vi "S2DS_Edit Channel Info.vi"(4 "error in":errorcluster, 5 "Array channel in":T1, 6 "Port list":T10, 7 "Use array inst?":bool) -> (0 "error out":errorcluster, 1 "OK?":bool, 2 "False channel (out)":string[][](array[string]), 3 "All channel parameters (out)":T2 {"Scan parameters"."Y data taking" items=["in both direction", "in up direction only", "in down direction only"]; "Scan parameters"."X data taking" items=["in both direction", "in up direction only", "in down direction only"]})   [LabVIEW 2025]
uses:
  TYPE DEFS/S2DS_DAC info new.ctl
  TYPE DEFS/S2DS_Single DC info.ctl
  TYPE DEFS/S2DS_RC info.ctl
  TYPE DEFS/S2DS_Single RC info.ctl
  TYPE DEFS/S2DS_WC info.ctl
  TYPE DEFS/S2DS_Single WC info.ctl
  TYPE DEFS/S2DS_Port lists.ctl
  TYPE DEFS/S2DS_All Channel Parameters.ctl
  TYPE DEFS/S2DS_Array Inst Info.ctl
  TYPE DEFS/S2DS_Sweep Info.ctl
panel:
  in  "Load config":bool
  in  "Save channel":bool
  in  "Tab Control":T11(tab)
  in  "Add  WC":bool
  in  "WC base unit":string caption="Unit"
  in  "Prefactor":string(combo)=" "
  in  "WC name":string caption="Name"
  in  "WC Factor":dbl=1.0 caption="Factor"
  in  "WC Present value":dbl caption="Present level"
  in  "WC instrument menu":string(combo) caption="Select instrument"
  in  "Clear WCs":bool
  out "WC info list":T3 caption="Channel info list"
  in  "Select WC":i32(ring) items=["A", "B"]
  in  "Replace WC":bool
  in  "Delete WC":bool
  in  "Enable":bool
  in  "RC name":string caption="Name"
  in  "RC instrument menu":string(combo) caption="Select instrument"
  in  "RC Amplification":dbl=1.0 caption="Factor"
  in  "RC unit":string caption="Unit"
  in  "Prefactor":string(combo)=" "
  in  "Add  RC":bool
  in  "Clear RCs":bool
  in  "Replace RC":bool
  in  "Select RC":i32(ring) items=["R"]
  in  "Delete RC":bool
  out "RC info list":T5 caption="Name            Unit          Instrument port  Total fact     Avg            Wait"
  in  "Enable 2":bool caption="Enable"
  in  "U":u16(ring) items=["Constant", "A", "B", "C"]
  in  "DC name":string caption="Name"
  in  "DC operation name":string(combo)="f*(u/v)" caption="Operation"
  in  "DC Factor":dbl=1.0 caption="Factor"
  in  "DC unit":string caption="Unit"
  in  "Add  DC":bool
  in  "DC constant":dbl=1.0 caption="Constant"
  in  "Clear DC":bool
  out "DC info list":T7 caption="Name              Unit          Operation               Factor & Constant         U         V"
  in  "V":u16(ring) items=["Constant", "A", "B", "C"]
  in  "Select DC":i32(ring) items=["C"]
  in  "Replace DC":bool
  in  "Delete DC":bool
  in  "Factor":dbl[](array[numeric])
  in  "Port names":string[](array[string])
  in  "Units":string[](array[string])
  in  "Units prefactor":string[](array[combo])
  in  "Cancel":bool
  in  "OK":bool
  # "Edit channel info"
  # "Name                    Unit            Instrument port      Total  factor    Present level"
  # "Typically, Total factor X Externa amplification = 1."
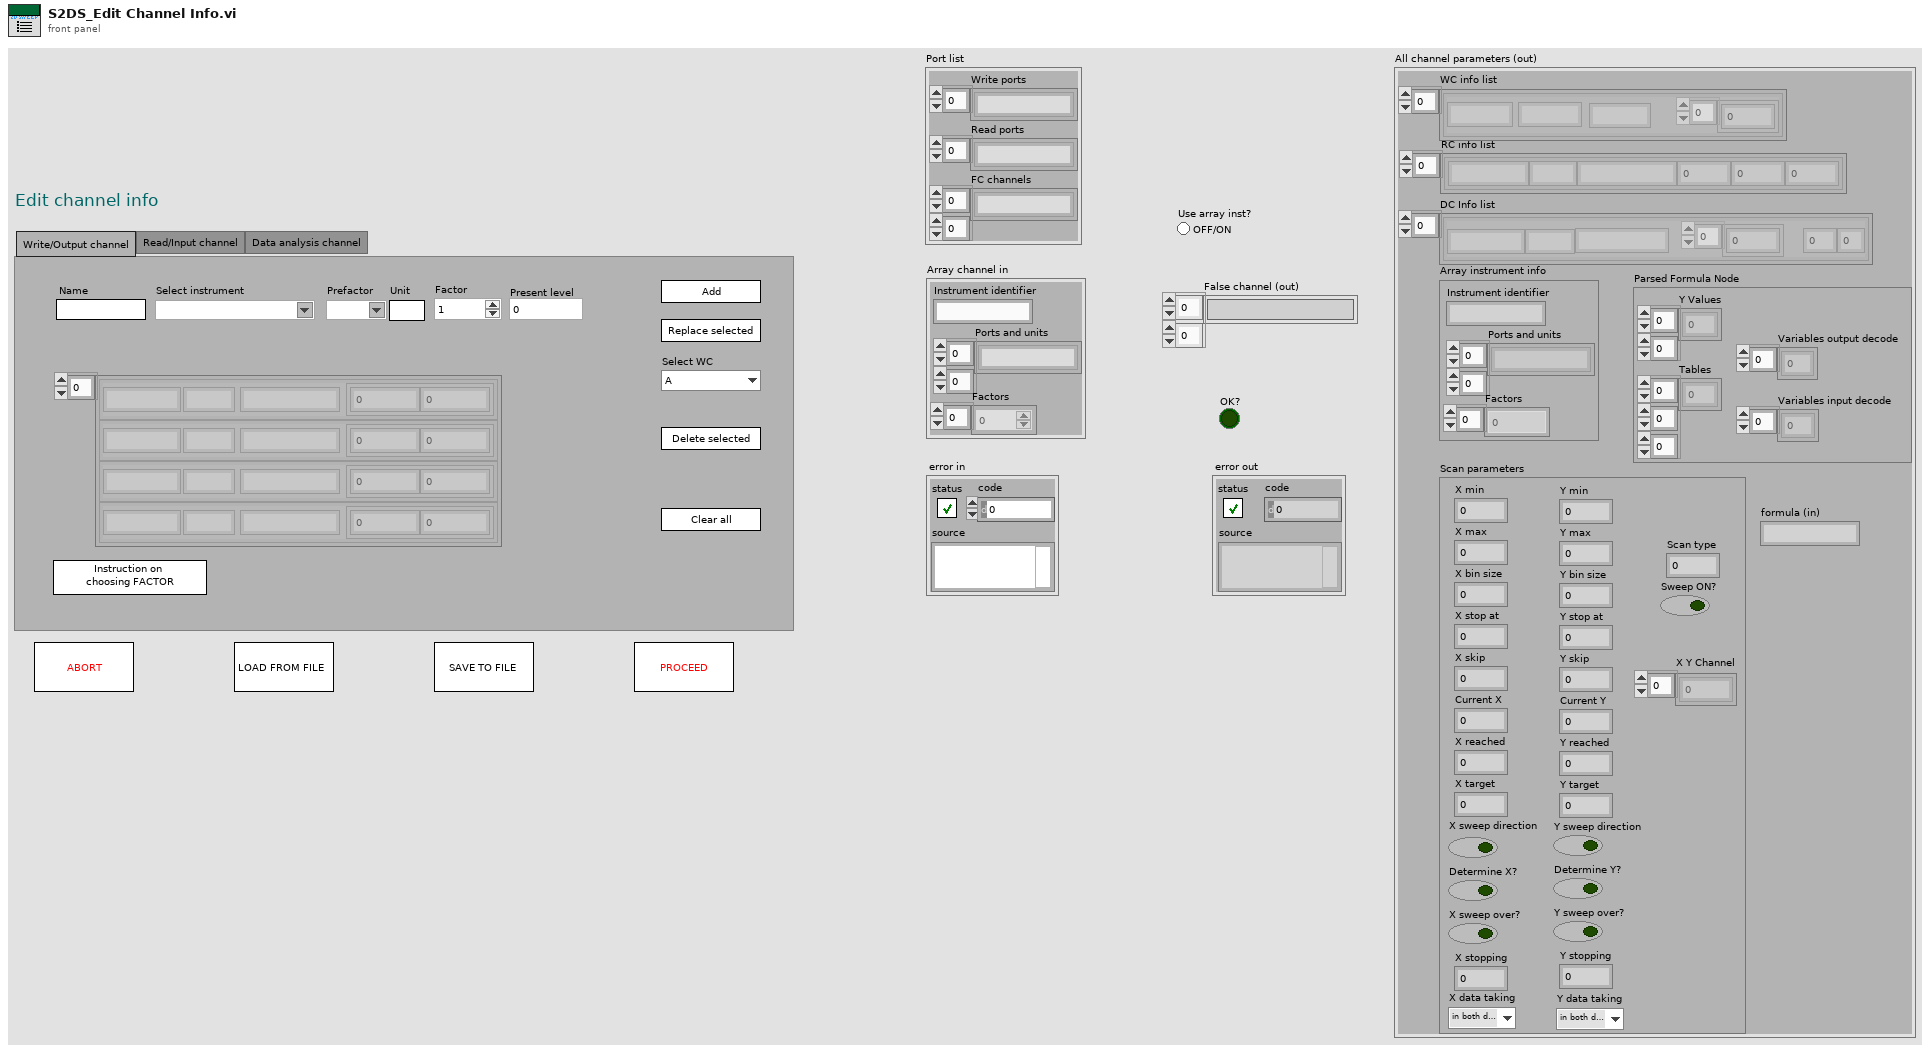
[diagram p1: front panel]
types:
  T1 = typedef "S2DS_Array Inst Info.ctl" = cluster{"Instrument identifier":string, "Ports and units":string[][], "Factors":dbl[]}
  T2 = typedef "S2DS_All Channel Parameters.ctl" = cluster{"WC info list":T3, "RC info list":T5, "DC Info list":T7, "Array instrument info":T1, "Scan parameters":T9, "Parsed Formula Node":cluster{"Y Values":dbl[][], "Tables":i32[][][], "Variables input decode":i32[], "Variables output decode":i32[]}, "formula (in)":string}
  T3 = typedef "S2DS_WC info.ctl" = T4[]
  T4 = typedef "S2DS_Single WC info.ctl" = cluster{"Instrument identifier":string, "Write channel parameters":dbl[], "Name":string, "Unit":string}
  T5 = typedef "S2DS_RC info.ctl" = T6[]
  T6 = typedef "S2DS_Single RC info.ctl" = cluster{"Instrument identifier":string, "Factor":dbl, "Averaging":i32, "Wait (ms)":i32, "Unit":string, "Name":string}
  T7 = typedef "S2DS_DAC info new.ctl" = T8[]
  T8 = typedef "S2DS_Single DC info.ctl" = cluster{"Operation identifier":string, "DC parameters":dbl[], "U":i32, "V":i32, "Name":string, "Unit":string}
  T9 = typedef "S2DS_Sweep Info.ctl" = cluster{"X min":ext, "X max":dbl, "Y min":dbl, "Y max":dbl, "X bin size":dbl, "Y bin size":dbl, "X stop at":dbl, "Y stop at":dbl, "X skip":u64, "Y skip":u64, "Current X":dbl, "Current Y":dbl, "X reached":i32, "Y reached":i32, "X target":dbl, "Y target":dbl, "Sweep ON?":bool, "X sweep direction":bool, "Y sweep direction":bool, "Determine X?":bool, "Determine Y?":bool, "X sweep over?":bool, "Y sweep over?":bool, "Scan type":i32, "X stopping":i32, "Y stopping":i32, "X Y Channel":u16[], "X data taking":u16, "Y data taking":u16}
  T10 = typedef "S2DS_Port lists.ctl" = cluster{"Write ports":string[], "Read ports":string[], "FC channels":string[][]}
  T11 = enum32{"Write/Output channel", "Read/Input channel", "Data analysis channel", "Array Output Channel"}
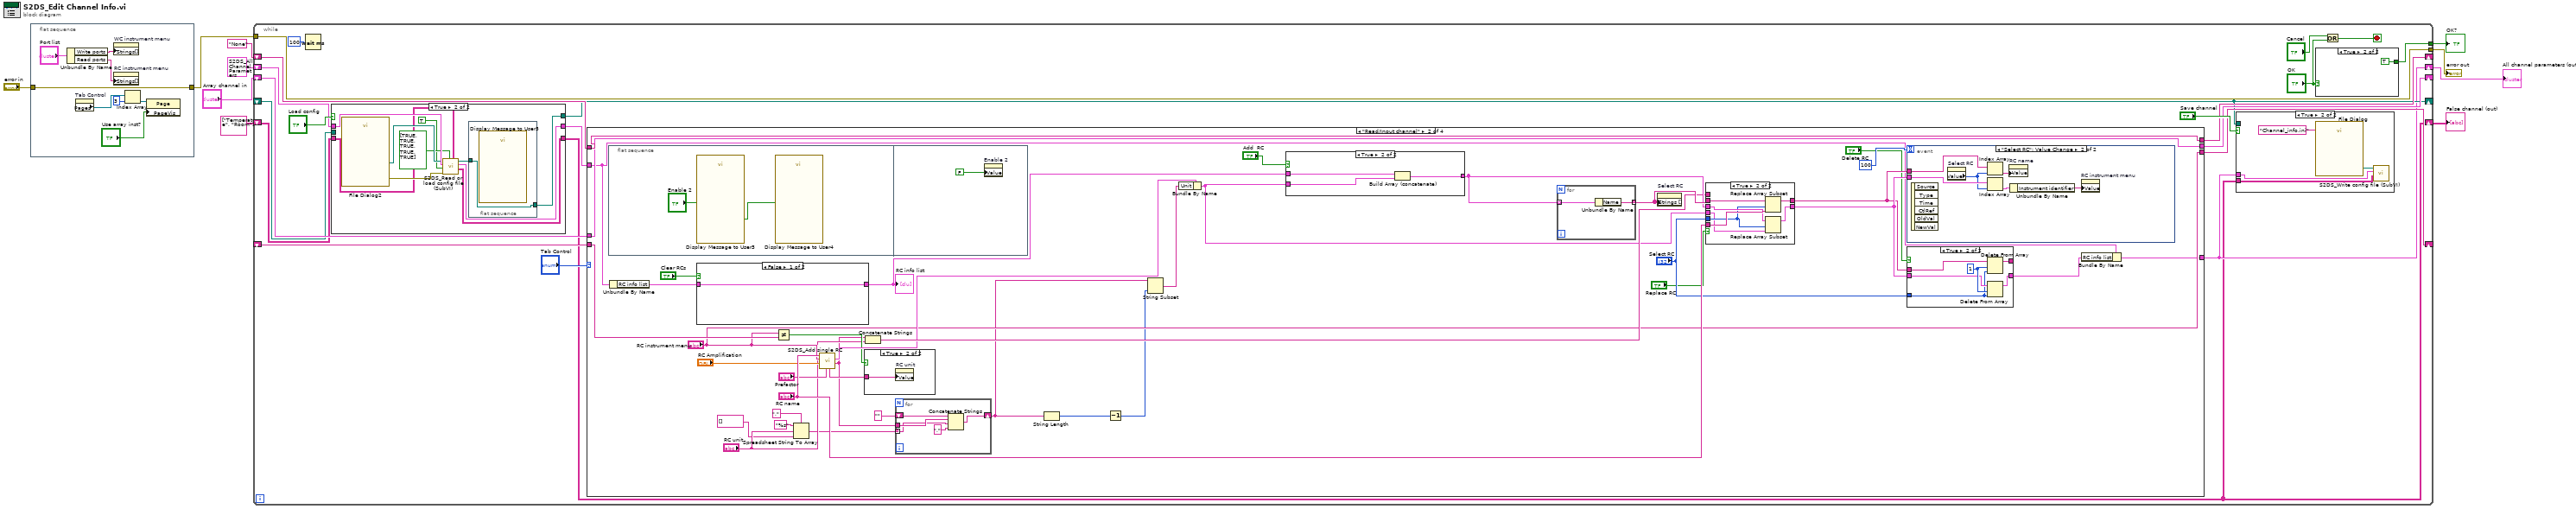
[diagram p0: block diagram]
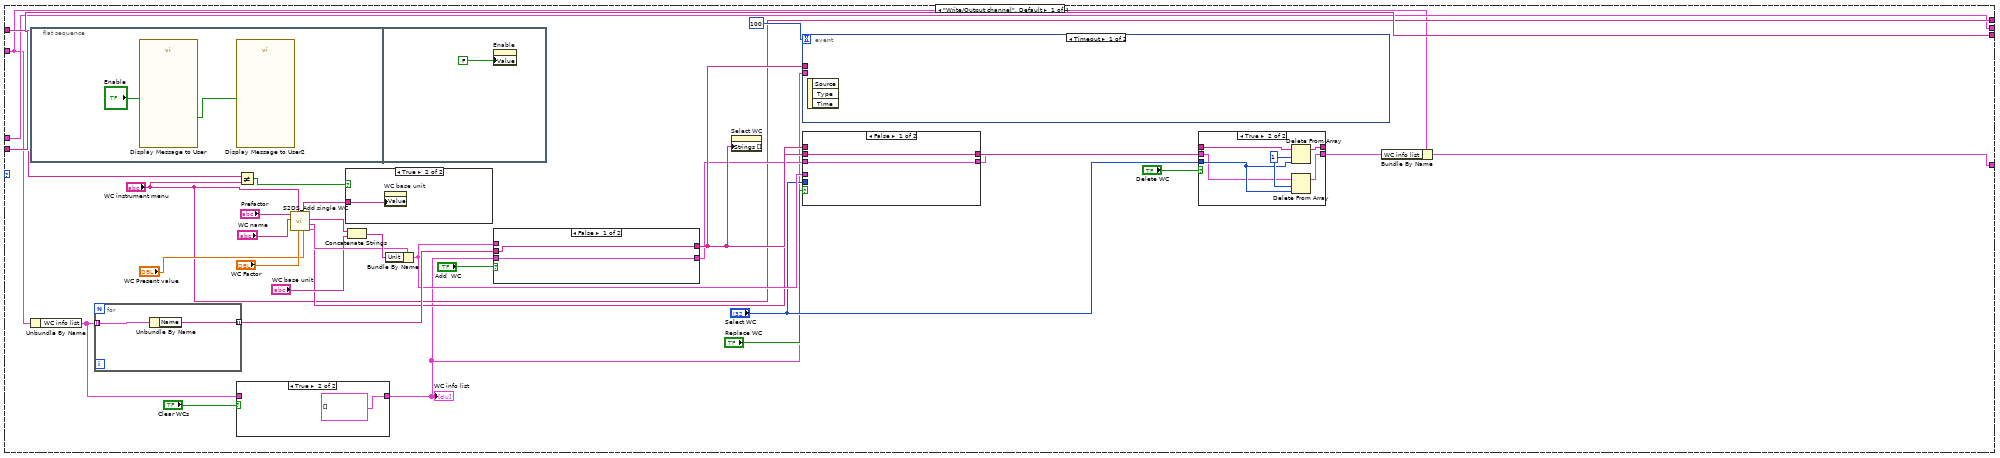
[diagram p2: hidden frame]
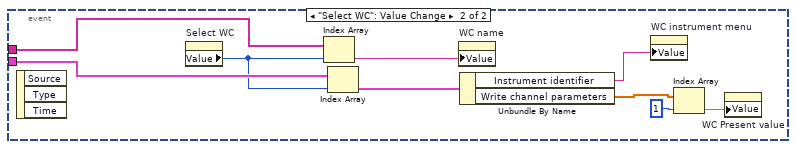
[diagram p3: hidden frame]
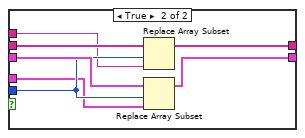
[diagram p6: hidden frame]
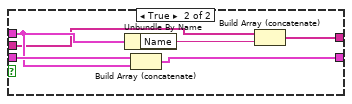
[diagram p7: hidden frame]
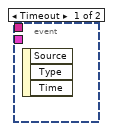
[diagram p9: hidden frame]
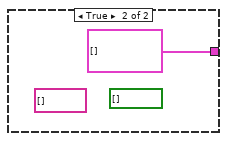
[diagram p14: hidden frame]
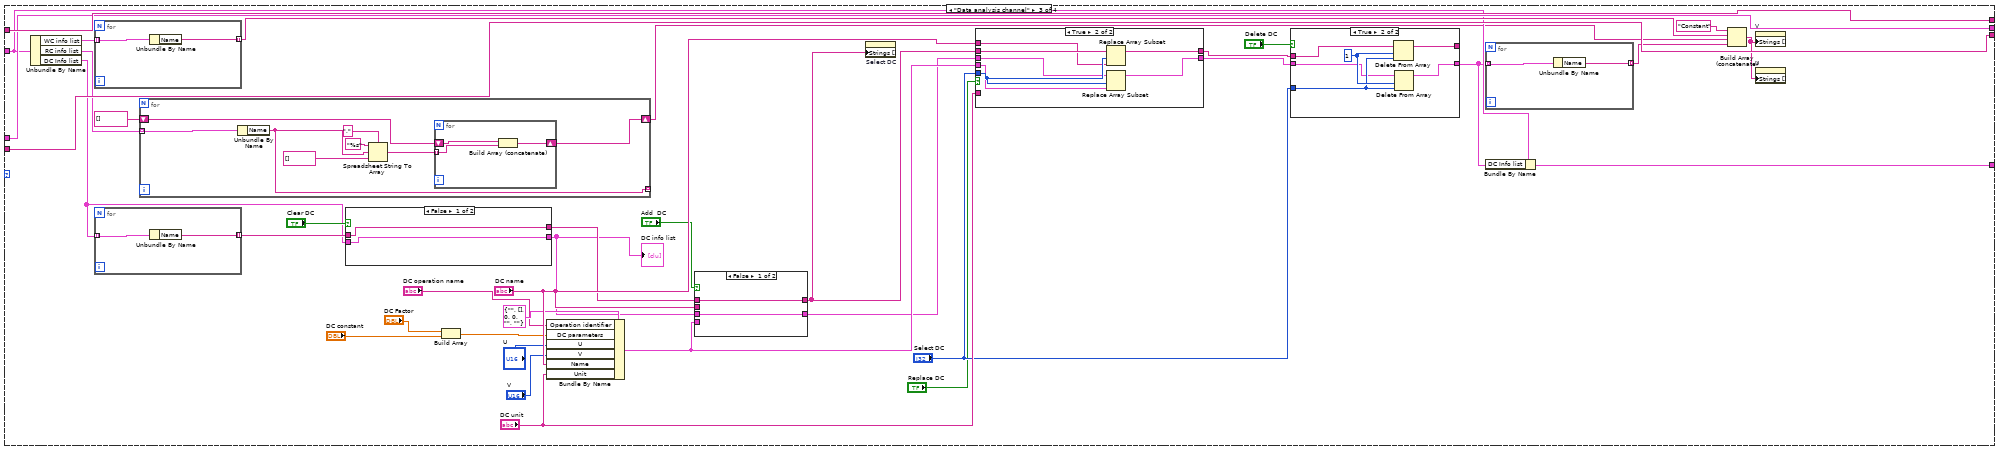
[diagram p15: hidden frame]
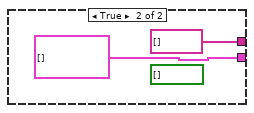
[diagram p18: hidden frame]
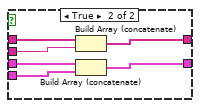
[diagram p19: hidden frame]
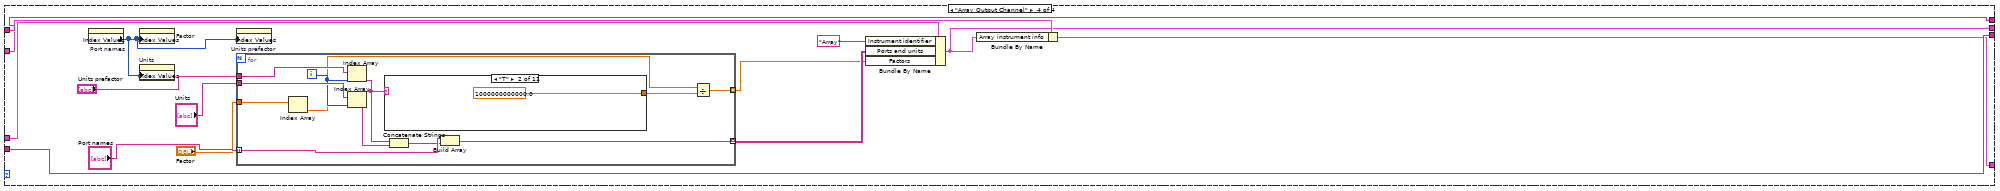
[diagram p20: hidden frame]
diagram:
  n1 = flat-sequence {
    tunnel: [w15] -> w8
    tunnel: "error in" -> [w15]
    frame #0 {
      n2 = Unbundle By Name("Port list") -> ("Write ports"=w17:string[], "Read ports"=w16:string[])
      n3 = property on="Tab Control" class="TabCtl (strict)"() -> ("Pages"=w12:refnum<vi>[])  [unwired: 2 in, 2 out]
      n4 = property on="WC instrument menu" class="CmbBox"("Strings[]"=w17) -> ()  [unwired: 2 in, 2 out]
      n5 = property on="RC instrument menu" class="CmbBox"("Strings[]"=w16) -> ()  [unwired: 2 in, 2 out]
      n6 = Index Array(array=w12, index=3) -> (element=w14:refnum<vi>)
      n7 = property class="Page"(reference=w14, "PageVis"="Use array inst?") -> ()  [unwired: 1 in, 2 out]
    }
  }
  n8 = while {
    tunnel: [w37] -> w6
    tunnel: w8 -> [w35]
    tunnel: [w35] -> w10
    shift-right: [w29] -> _
    shift-left: "None" ("WC name") -> [w28]
    shift-right: [w30] -> _
    shift-left: _ -> [w31]
    shift-right: [w27] -> _
    shift-left: "Array channel in" -> [w26]
    shift-right: [w24] -> _
    shift-left: _ -> [w25]
    shift-right: [w21] -> w4
    shift-left: T2 {"WC info list"=[], "RC info list"=[], "DC Info list"=[], "Array instrument info"={"Instrument identifier"="", "Ports and units"=[], "Factors"=[]}, "Scan parameters"={"X min"=0.0, "X max"=1.0, "Y min"=0.0, "Y max"=1.0, "X bin size"=0.001, "Y bin size"=0.001, "X stop at"=0.0, "Y stop at"=0.0, "X skip"=0, "Y skip"=0, "Current X"=0.0, "Current Y"=0.0, "X reached"=0, "Y reached"=0, "X target"=0.0, "Y target"=0.0, "Sweep ON?"=FALSE, "X sweep direction"=FALSE, "Y sweep direction"=FALSE, "Determine X?"=FALSE, "Determine Y?"=FALSE, "X sweep over?"=FALSE, "Y sweep over?"=FALSE, "Scan type"=0, "X stopping"=0, "Y stopping"=0, "X Y Channel"=[], "X data taking"=0, "Y data taking"=0}, "Parsed Formula Node"={"Y Values"=[], "Tables"=[], "Variables input decode"=[], "Variables output decode"=[]}, "formula (in)"=""} ("All channel parameters (in)") -> [w23]
    shift-right: [w19] -> w1
    shift-left: string[][] [["Temperature", "Room"]] ("False channel (out)") -> [w20]
    stop <- w40 stop-if-true
    n9 = Wait (ms)(milliseconds to wait=u32 100) -> ()  [unwired: 1 out]
    n10 = case shown="True" "Load config" {
      tunnel: [w315 w317] -> w24
      tunnel: w25 -> [w315 _]
      tunnel: w23 -> [w314 w325]
      tunnel: [w314 w324] -> w22
      tunnel: [w313 w318] -> w19
      tunnel: w20 -> [w313 w319]
      frame False {
      }
      frame True {
        n11 = call "File Dialog2"() -> ("selected path"=w323:path, "error out"=w322:errorcluster)  [unwired: 12 in, 2 out]
        n12 = call "S2DS_Read or load config file (SubVI).vi"("False channel (in)"=w319, "Loading information in"=bool[] [TRUE, TRUE, TRUE, TRUE, TRUE], "error in (no error)"=w322, "Update present value?"=TRUE ("Accept target?"), "All channel parameters (in)"=w325, "selected path"=w323) -> ("False channel (out)"=w318:string[][], "All channel parameters (out)"=w324:T2, "file path"=w316:path)  [unwired: 2 in, 1 out]
        n13 = flat-sequence {
          tunnel: [w326] -> w317
          tunnel: w316 -> [w326]
          frame #0 {
            n14 = call "Display Message to User5"() -> ()  [unwired: 10 in, 2 out]
          }
        }
      }
    }
    n15 = case shown="\"Read/Input channel\"" "Tab Control" {
      tunnel: w31 -> [w72 w134 w229 w289]
      tunnel: [w72 "RC instrument menu" w229 w289] -> w30
      tunnel: ["WC instrument menu" w132 w206 w288] -> w29
      tunnel: w28 -> [w47 w132 w206 w288]
      tunnel: [w45 w131 w205 w280] -> w27
      tunnel: w26 -> [w45 w131 w205 w284]
      tunnel: w22 -> [w43 w129 w197 w281]
      tunnel: [w41 w127 w195 w279] -> w21
      frame "Write/Output channel", Default {
        n16 = flat-sequence {
          frame #0 {
            n17 = call "Display Message to User"("Enable"="Enable") -> ("Not understood"=w73:bool)  [unwired: 9 in, 1 out]
            n18 = call "Display Message to User2"("Enable"=w73) -> ()  [unwired: 9 in, 2 out]
          }
          frame #1 {
            n19 = property on="Enable" class="Bool (strict)"("Value"=FALSE ("Enable")) -> ()  [unwired: 2 in, 2 out]
          }
        }
        n20 = Unbundle By Name(w43) -> ("WC info list"=w44:T3)
        n21 = for {
          tunnel: w44 -> [w77] mode=indexing
          tunnel: [w76] -> w71 mode=indexing
          n22 = Unbundle By Name(w77) -> ("Name"=w76:string)
        }
        n23 = case shown="True" "Clear WCs" {
          tunnel: w44 -> [w113 _]
          tunnel: [w113 T3 [] ("WC Info list")] -> w46
          frame False {
          }
          frame True {
          }
        }
        "WC info list" <- w46
        n24 = Not Equal?(x=w47, y="WC instrument menu") -> (x != y?=w63:bool)
        n25 = call "S2DS_Add single WC.vi"("WC Present value"="WC Present value", "WC Factor"="WC Factor", "WC instrument menu"="WC instrument menu", "WC name in"="WC name", "prefix"="Prefactor") -> ("Write channel info"=w67:T4, "WC name out"=w56:string, "Prefix"=w61:string, "Base unit"=w64:string)  [unwired: 3 in]
        n26 = case shown="True" w63 {
          tunnel: w64 -> [_ w87]
          frame False {
          }
          frame True {
            n27 = property on="WC base unit" class="Str"("Value"=w87) -> ()  [unwired: 2 in, 2 out]
          }
        }
        n28 = Concatenate Strings(w61, "WC base unit") -> (w69:string)
        n29 = Bundle By Name(cluster=w67, "Unit"=w69) -> (w68:T4)
        n30 = case shown="False" "Add  WC" {
          tunnel: w46 -> [w106 w112]
          tunnel: [w106 w111] -> w55
          tunnel: w68 -> [_ w109]
          tunnel: [w105 w110] -> w70
          tunnel: w71 -> [w105 w107]
          frame False {
          }
          frame True {
            n31 = Unbundle By Name(w109) -> ("Name"=w108:string)
            n32 = Build Array (concatenate)(w112, w109) -> (w111:T3)
            n33 = Build Array (concatenate)(w107, w108) -> (w110:string[])
          }
        }
        n34 = property on="Select WC" class="Ring (strict)"("Strings []"=w70) -> ()  [unwired: 2 in, 2 out]
        n35 = event shown="[0] Timeout" {
          selector: _ -> [_ _]
          dyn-events: _ -> [_ _]
          timeout: 100 -> [_ _]
          tunnel: w46 -> [_ w86]
          tunnel: w70 -> [_ w83]
          event Timeout {
            n36 = event-data() -> ()  [unwired: 1 in, 3 out]
          }
          event "Select WC": Value Change {
            n37 = event-data() -> ()  [unwired: 1 in, 3 out]
            n38 = property on="Select WC" class="Ring (strict)"() -> ("Value"=w78:i32)  [unwired: 2 in, 2 out]
            n39 = Index Array(array=w83, index=w78) -> (element=w82:string)
            n40 = Index Array(array=w86, index=w78) -> (element=w85:T4)
            n41 = property on="WC name" class="Str"("Value"=w82) -> ()  [unwired: 2 in, 2 out]
            n42 = Unbundle By Name(w85) -> ("Instrument identifier"=w84:string, "Write channel parameters"=w81:dbl[])
            n43 = property on="WC instrument menu" class="CmbBox"("Value"=w84) -> ()  [unwired: 2 in, 2 out]
            n44 = Index Array(array=w81, index=1) -> (element=w79:dbl)
            n45 = property on="WC Present value" class="DigNum (strict)"("Value"=w79) -> ()  [unwired: 2 in, 2 out]
          }
        }
        n46 = case shown="False" "Replace WC" {
          tunnel: w55 -> [w97 w104]
          tunnel: [w97 w103] -> w57
          tunnel: "Select WC" -> [_ w102]
          tunnel: w68 -> [_ w101]
          tunnel: w70 -> [w96 w100]
          tunnel: [w96 w99] -> w58
          tunnel: w56 -> [_ w98]
          frame False {
          }
          frame True {
            n47 = Replace Array Subset(array=w100, new element=w98, index=w102) -> (w99:string[])
            n48 = Replace Array Subset(array=w104, new element=w101, index=w102) -> (w103:T3)
          }
        }
        n49 = case shown="True" "Delete WC" {
          tunnel: "Select WC" -> [_ w94]
          tunnel: w57 -> [w89 w93]
          tunnel: [w89 w92] -> w42
          tunnel: w58 -> [w88 w91]
          tunnel: [w88 w90] -> _
          frame False {
          }
          frame True {
            w95 = 1 ("length")
            n50 = Delete From Array(array=w91, length=w95, index=w94) -> (array with subset deleted=w90:string[])  [unwired: 1 out]
            n51 = Delete From Array(array=w93, length=w95, index=w94) -> (array with subset deleted=w92:T3)  [unwired: 1 out]
          }
        }
        n52 = Bundle By Name(cluster=w43, "WC info list"=w42) -> (w41:T2)
      }
      frame "Read/Input channel" {
        n53 = flat-sequence {
          frame #0 {
            n54 = call "Display Message to User3"("Enable"="Enable 2") -> ("Not understood"=w158:bool)  [unwired: 9 in, 1 out]
            n55 = call "Display Message to User4"("Enable"=w158) -> ()  [unwired: 9 in, 2 out]
          }
          frame #1 {
            n56 = property on="Enable 2" class="Bool (strict)"("Value"=FALSE ("Enable")) -> ()  [unwired: 2 in, 2 out]
          }
        }
        n57 = Unbundle By Name(w129) -> ("RC info list"=w130:T5)
        n58 = case shown="False" "Clear RCs" {
          tunnel: w130 -> [w191 _]
          tunnel: [w191 T5 [] ("RC Info list")] -> w137
          frame False {
          }
          frame True {
            (unwired) bool[] [] ("WC Save info")
            (unwired) string[] [] ("WC names")
          }
        }
        "RC info list" <- w137
        n59 = Not Equal?(x="RC instrument menu", y=w134) -> (x != y?=w143:bool)
        n60 = Spreadsheet String To Array(delimiter (Tab)=",", format string="%s", spreadsheet string="RC unit", array type (2D Dbl)=string[] []) -> (array=w121:string[])
        n61 = call "S2DS_Add single RC.vi"("prefix in"="Prefactor", "RC Factor"="RC Amplification", "RC instrument menu"="RC instrument menu", "RC name in"="RC name") -> ("Prefix unit"=w119:string, "Read channel info"=w148:T6, "Base unit"=w144:string)  [unwired: 5 in]
        n62 = case shown="True" w143 {
          tunnel: w144 -> [_ w169]
          frame False {
          }
          frame True {
            n63 = property on="RC unit" class="Str"("Value"=w169) -> ()  [unwired: 2 in, 2 out]
          }
        }
        n64 = Concatenate Strings(w119, "RC unit") -> (w149:string)
        n65 = for {
          tunnel: w121 -> [w154] mode=indexing
          shift-right: [w156] -> w118
          shift-left: "" -> [w157]
          tunnel: w119 -> [w155]
          n66 = Concatenate Strings(w157, w155, w154, "," ("string")) -> (w156:string)
        }
        n67 = String Length(string=w118) -> (length=w117:i32)
        n68 = Decrement(x=w117) -> (x-1=w116:i32)
        n69 = String Subset(string=w118, length (rest)=w116) -> (substring=w115:string)  [unwired: 1 in]
        n70 = Bundle By Name(cluster=w148, "Unit"=w115) -> (w126:T6)
        n71 = case shown="True" "Add  RC" {
          tunnel: w137 -> [w187 w190]
          tunnel: [w187 w189] -> w150
          tunnel: w126 -> [_ w188]
          frame False {
          }
          frame True {
            n72 = Build Array (concatenate)(w190, w188) -> (w189:T5)
          }
        }
        n73 = for {
          tunnel: w150 -> [w162] mode=indexing
          tunnel: [w161] -> w151 mode=indexing
          n74 = Unbundle By Name(w162) -> ("Name"=w161:string)
        }
        n75 = property on="Select RC" class="Ring (strict)"("Strings []"=w151) -> ()  [unwired: 2 in, 2 out]
        n76 = case shown="True" "Replace RC" {
          tunnel: [w179 w184] -> w146
          tunnel: w151 -> [w179 w186]
          tunnel: [w178 w182] -> w147
          tunnel: w150 -> [w178 w183]
          tunnel: "Select RC" -> [_ w181]
          tunnel: "RC name" -> [_ w185]
          tunnel: w149 -> [_ _]
          tunnel: w126 -> [_ w180]
          frame False {
          }
          frame True {
            n77 = Replace Array Subset(array=w186, new element=w185, index=w181) -> (w184:string[])
            n78 = Replace Array Subset(array=w183, new element=w180, index=w181) -> (w182:T5)
          }
        }
        n79 = event shown="[1] \"Select RC\": Value Change" {
          selector: _ -> [_ _]
          dyn-events: _ -> [_ _]
          timeout: 100 -> [_ _]
          tunnel: w146 -> [_ w165]
          tunnel: w147 -> [_ w168]
          event Timeout {
            n80 = event-data() -> ()  [unwired: 1 in, 3 out]
          }
          event "Select RC": Value Change {
            n81 = event-data() -> ()  [unwired: 1 in, 6 out]
            n82 = property on="Select RC" class="Ring (strict)"() -> ("Value"=w163:i32)  [unwired: 2 in, 2 out]
            n83 = Index Array(array=w165, index=w163) -> (element=w164:string)
            n84 = Index Array(array=w168, index=w163) -> (element=w167:T6)
            n85 = property on="RC name" class="Str"("Value"=w164) -> ()  [unwired: 2 in, 2 out]
            n86 = Unbundle By Name(w167) -> ("Instrument identifier"=w166:string)
            n87 = property on="RC instrument menu" class="CmbBox"("Value"=w166) -> ()  [unwired: 2 in, 2 out]
          }
        }
        n88 = case shown="True" "Delete RC" {
          tunnel: w146 -> [w171 w177]
          tunnel: [w171 w176] -> _
          tunnel: "Select RC" -> [_ w172]
          tunnel: w147 -> [w170 w174]
          tunnel: [w170 w173] -> w128
          frame False {
          }
          frame True {
            w175 = 1 ("length")
            n89 = Delete From Array(array=w177, length=w175, index=w172) -> (array with subset deleted=w176:string[])  [unwired: 1 out]
            n90 = Delete From Array(array=w174, length=w175, index=w172) -> (array with subset deleted=w173:T5)  [unwired: 1 out]
          }
        }
        n91 = Bundle By Name(cluster=w129, "RC info list"=w128) -> (w127:T2)
      }
      frame "Data analysis channel" {
        n92 = Unbundle By Name(w197) -> ("WC info list"=w200:T3, "RC info list"=w199:T5, "DC Info list"=w198:T7)
        n93 = for {
          tunnel: w200 -> [w244] mode=indexing
          tunnel: [w243] -> w202 mode=indexing
          n94 = Unbundle By Name(w244) -> ("Name"=w243:string)
        }
        n95 = for {
          tunnel: w198 -> [w246] mode=indexing
          tunnel: [w245] -> w228 mode=indexing
          n96 = Unbundle By Name(w246) -> ("Name"=w245:string)
        }
        n97 = for {
          tunnel: w199 -> [w239] mode=indexing
          tunnel: [w232] -> _ mode=indexing
          shift-right: [w235] -> w193
          shift-left: string[] [] -> [w236]
          n98 = Unbundle By Name(w239) -> ("Name"=w232:string)
          n99 = Spreadsheet String To Array(delimiter (Tab)=",", format string="%s" ("spreadsheet string"), spreadsheet string=w232, array type (2D Dbl)=string[] []) -> (array=w237:string[])
          n100 = for {
            tunnel: w237 -> [w241] mode=indexing
            shift-right: [w240] -> w235
            shift-left: w236 -> [w242]
            n101 = Build Array (concatenate)(w242, w241) -> (w240:string[])
          }
        }
        n102 = case shown="False" "Clear DC" {
          tunnel: w198 -> [w265 _]
          tunnel: [w265 T7 [] ("DC Info list")] -> w209
          tunnel: w228 -> [w264 _]
          tunnel: [w264 string[] [] ("WC names")] -> w210
          frame False {
          }
          frame True {
            (unwired) bool[] [] ("WC Save info")
          }
        }
        "DC info list" <- w209
        n103 = Build Array("DC Factor", "DC constant") -> (w217:dbl[])
        n104 = Bundle By Name(cluster=T8 {"Operation identifier"="", "DC parameters"=[], "U"=0, "V"=0, "Name"="", "Unit"=""} ("Data analysis channel info"), "Operation identifier"="DC operation name", "DC parameters"=w217, "U"="U", "V"="V", "Name"="DC name", "Unit"="DC unit") -> (w220:T8)
        n105 = case shown="False" "Add  DC" {
          tunnel: [w269 w274] -> w213
          tunnel: w209 -> [w269 w275]
          tunnel: [w268 w272] -> w212
          tunnel: w210 -> [w268 w273]
          tunnel: "DC name" -> [_ w271]
          tunnel: w220 -> [_ w270]
          frame False {
          }
          frame True {
            n106 = Build Array (concatenate)(w273, w271) -> (w272:string[])
            n107 = Build Array (concatenate)(w275, w270) -> (w274:T7)
          }
        }
        n108 = property on="Select DC" class="Ring (strict)"("Strings []"=w212) -> ()  [unwired: 2 in, 2 out]
        n109 = case shown="True" "Replace DC" {
          tunnel: "Select DC" -> [_ w263]
          tunnel: w212 -> [w256 w262]
          tunnel: [w256 w261] -> w224
          tunnel: "DC name" -> [_ w260]
          tunnel: "DC unit" -> [_ _]
          tunnel: w213 -> [w255 w259]
          tunnel: [w255 w258] -> w223
          tunnel: w220 -> [_ w257]
          frame False {
          }
          frame True {
            n110 = Replace Array Subset(array=w262, new element=w260, index=w263) -> (w261:string[])
            n111 = Replace Array Subset(array=w259, new element=w257, index=w263) -> (w258:T7)
          }
        }
        n112 = case shown="True" "Delete DC" {
          tunnel: "Select DC" -> [_ w253]
          tunnel: w223 -> [w248 w252]
          tunnel: [w248 w251] -> w196
          tunnel: w224 -> [w247 w250]
          tunnel: [w247 w249] -> _
          frame False {
          }
          frame True {
            w254 = 1 ("length")
            n113 = Delete From Array(array=w250, length=w254, index=w253) -> (array with subset deleted=w249:string[])  [unwired: 1 out]
            n114 = Delete From Array(array=w252, length=w254, index=w253) -> (array with subset deleted=w251:T7)  [unwired: 1 out]
          }
        }
        n115 = for {
          tunnel: w196 -> [w231] mode=indexing
          tunnel: [w230] -> w201 mode=indexing
          n116 = Unbundle By Name(w231) -> ("Name"=w230:string)
        }
        n117 = Bundle By Name(cluster=w197, "DC Info list"=w196) -> (w195:T2)
        n118 = Build Array (concatenate)("Constant", w202, w193, w201) -> (w204:string[])
        n119 = property on="V" class="Ring (strict)"("Strings []"=w204) -> ()  [unwired: 2 in, 2 out]
        n120 = property on="U" class="Ring (strict)"("Strings []"=w204) -> ()  [unwired: 2 in, 2 out]
      }
      frame "Array Output Channel" {
        n121 = property on="Port names" class="Arr (strict)"() -> ("Index Values"=w287:u32[])  [unwired: 2 in, 2 out]
        n122 = property on="Factor" class="Arr (strict)"("Index Values"=w287) -> ()  [unwired: 2 in, 2 out]
        n123 = property on="Units" class="Arr (strict)"("Index Values"=w287) -> ()  [unwired: 2 in, 2 out]
        n124 = property on="Units prefactor" class="Arr (strict)"("Index Values"=w287) -> ()  [unwired: 2 in, 2 out]
        n125 = for {
          tunnel: "Units prefactor" -> [w293]
          tunnel: [w300] -> w278 mode=indexing
          tunnel: "Units" -> [w296]
          tunnel: [w297] -> w286 mode=indexing
          tunnel: "Port names" -> [w299] mode=indexing
          tunnel: "Factor" -> [w291]
          i -> [w292]
          n126 = Index Array(array=w291) -> (element=w290:dbl)  [unwired: 1 in]
          n127 = Index Array(array=w293, index=w292) -> (element=w294:string)
          n128 = Index Array(array=w296, index=w292) -> (element=w295:string)
          n129 = case shown="\"T\"" w294 {
            tunnel: [1.0 1000000000000.0 1000000000.0 1000000.0 1000.0 0.001 1e-06 1e-09 1e-12 1e-15 1e-18] -> w301
            frame "False", Default {
            }
            frame "T" {
            }
            frame "G" {
            }
            frame "M" {
            }
            frame "k" {
            }
            frame "m" {
            }
            frame "u" {
            }
            frame "n" {
            }
            frame "p" {
            }
            frame "f" {
            }
            frame "a" {
            }
          }
          n130 = Concatenate Strings(w294, w295) -> (w298:string)
          n131 = Build Array(w299, w298) -> (w297:string[])
          n132 = Divide(x=w290, y=w301) -> (x/y=w300:dbl)
        }
        n133 = Bundle By Name(cluster=w284, "Instrument identifier"="Array", "Ports and units"=w286, "Factors"=w278) -> (w280:T1)
        n134 = Bundle By Name(cluster=w281, "Array instrument info"=w280) -> (w279:T2)
      }
    }
    n135 = case shown="True" "Save channel" {
      tunnel: w24 -> [_ _]
      tunnel: w21 -> [_ w329]
      tunnel: w19 -> [_ w327]
      frame False {
      }
      frame True {
        n136 = call "File Dialog"("default name"="Channel_info.ini") -> ("selected path"=w328:path)  [unwired: 11 in, 3 out]
        n137 = call "S2DS_Write config file (SubVI).vi"("False channel"=w327, "All channel parameters"=w329, "file path (use dialog)"=w328) -> ()  [unwired: 7 in, 2 out]
      }
    }
    n138 = case shown="True" "OK" {
      tunnel: [FALSE TRUE] -> w37
      frame False {
      }
      frame True {
      }
    }
    n139 = Or(x="Cancel", y="OK") -> (x .or. y?=w40:bool)
  }
  "OK?" <- w6
  "error out" <- w10
  "All channel parameters (out)" <- w4
  "False channel (out)" <- w1
